vi "Active Plugins.vi"(8 "error in (no error)":errorcluster, 11 "Framework in":refnum<class "Framework.lvclass">) -> (0 "error out":errorcluster, 3 "Framework out":refnum<class "Framework.lvclass">)   [LabVIEW 2017]
uses:
  Framework.lvclass
  Plugin/Plugin.lvclass
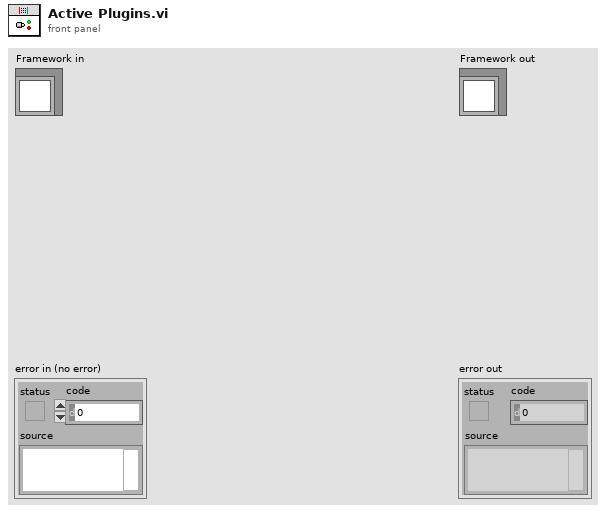
[diagram p1: front panel]
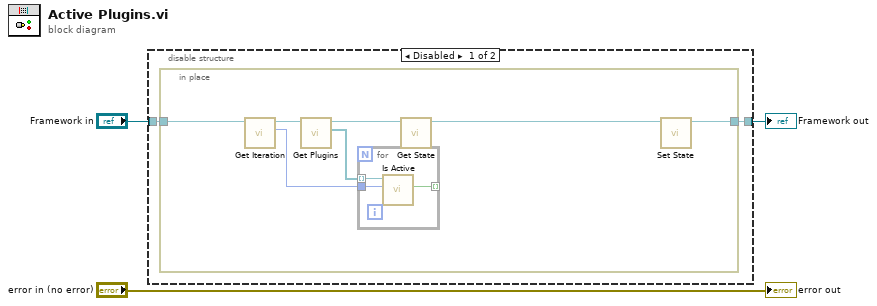
[diagram p0: block diagram]
diagram:
  n1 = disable-structure shown="Disabled" {
    disable-tunnel: [w5 w16] -> w3
    disable-tunnel: "Framework in" -> [w4 w16]
    frame Disabled {
      n2 = in-place {
        in-place-border: [w11] -> w5
        in-place-border: w4 -> [w9]
        n3 = call "Get Iteration.vi"("Framework in"=w9) -> ("iteration"=w6:u64, "Framework out"=w8:refnum<class "Framework.lvclass">)  [unwired: 9 in]
        n4 = call "Get Plugins.vi"("Framework in"=w8) -> ("Plugins"=w7:refnum<class "Plugin.lvclass">[], "Framework out"=w10:refnum<class "Framework.lvclass">)  [unwired: 9 in]
        n5 = for {
          tunnel: w7 -> [w15] mode=indexing
          tunnel: [w14] -> _ mode=indexing
          tunnel: w6 -> [w13]
          n6 = call "Is Active.vi"("cycle count"=w13, "Plugin in"=w15) -> ("active this cycle?"=w14:bool)  [unwired: 8 in, 1 out]
        }
        n7 = call "Get State.vi"("Framework in"=w10) -> ("Framework out"=w12:refnum<class "Framework.lvclass">)  [unwired: 9 in, 1 out]
        n8 = call "Set State.vi"("Framework in"=w12) -> ("Framework out"=w11:refnum<class "Framework.lvclass">)  [unwired: 10 in]
      }
    }
    frame Enabled {
    }
  }
  "Framework out" <- w3
  "error out" <- "error in (no error)"
